vi "Read Data.vi"(8 "error in (no error)":errorcluster, 11 "Cryomagnetics Power Supply in":refnum<class "Cryomagnetics Power Supply.lvclass">) -> (0 "error out":errorcluster, 2 "Data":waveform(dbl)[](array[waveform]), 3 "Cryomagnetics Power Supply out":refnum<class "Cryomagnetics Power Supply.lvclass">)   [LabVIEW 2015, in "Cryomagnetics Power Supply.lvclass"]
uses:
  Cryomagnetics Power Supply.lvclass
  Instrument/Instrument.lvclass
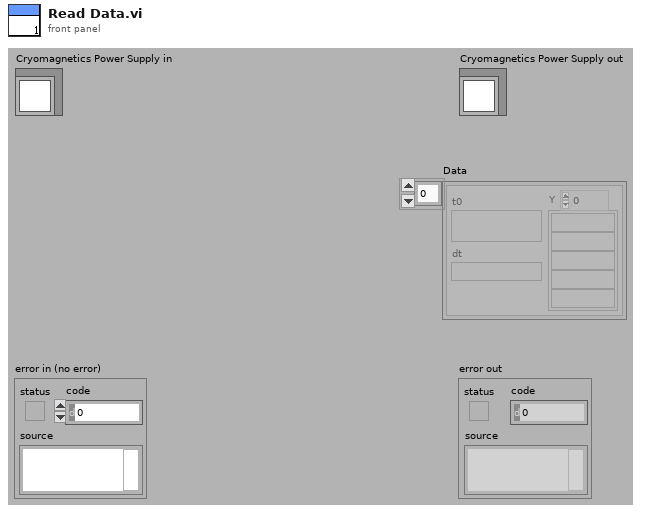
[diagram p1: front panel]
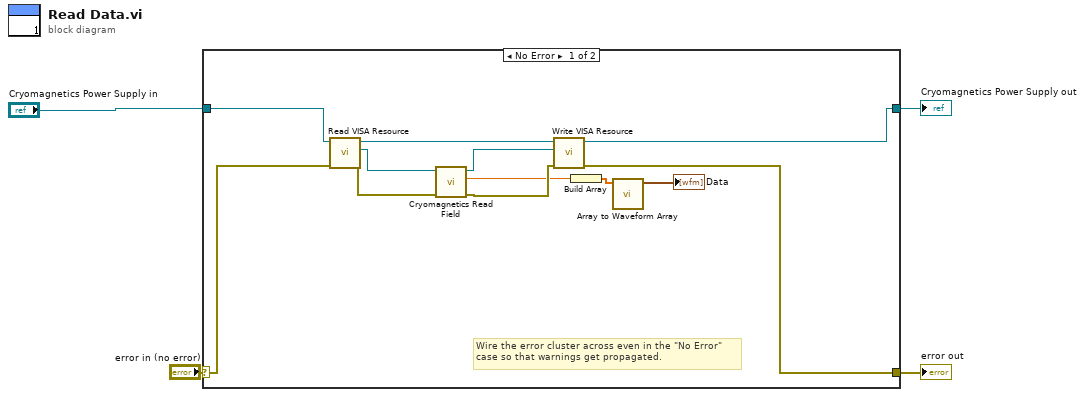
[diagram p0: block diagram]
diagram:
  n1 = case shown="No Error" "error in (no error)" {
    selector: "error in (no error)" -> [w5 w18]
    tunnel: [w6 w18] -> w3
    tunnel: [w7 w17] -> w1
    tunnel: "Cryomagnetics Power Supply in" -> [w8 w17]
    frame No Error {
      # "Wire the error cluster across even in the \"No Error\"\ncase so that warnings get propagated."
      n2 = call "Read VISA Resource.vi"("error in (no error)"=w5, "Instrument.lvclass in"=w8) -> ("error out"=w13:errorcluster, "VISA Resource"=w15:refnum<visa-resource-name>, "Instrument.lvclass out"=w16:refnum<class "Cryomagnetics Power Supply.lvclass">)  [unwired: 7 out]
      n3 = call "Cryomagnetics Read Field.vi"("error in (no error)"=w13, "VISA resource name"=w15) -> ("error out"=w12:errorcluster, "Field"=w11:dbl, "VISA Resource Name Out"=w14:refnum<visa-resource-name>)  [unwired: 6 in, 1 out]
      n4 = call "Write VISA Resource.vi"("error in (no error)"=w12, "VISA Resource"=w14, "Instrument.lvclass in"=w16) -> ("error out"=w6:errorcluster, "Instrument.lvclass out"=w7:refnum<class "Cryomagnetics Power Supply.lvclass">)  [unwired: 7 out]
      n5 = Build Array(w11) -> (w10:dbl[])
      n6 = call "Array to Waveform Array.vi"("Array"=w10) -> ("Waveform"=→"Data":waveform(dbl)[])  [unwired: 10 in]
    }
    frame Error {
    }
  }
  "error out" <- w3
  "Cryomagnetics Power Supply out" <- w1
